vi "LCR_development_test.vi"() -> ()   [LabVIEW 2018]
uses:
  InstrControl/LCRControl/LCRControl.lvclass
  InstrControl/InstrControl.lvclass
panel:
  out "Resistance in Ohm":dbl
  out "Capacitance in pF":dbl
  out "Instrument name OUT":string
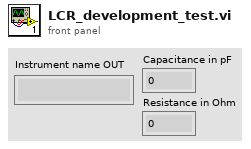
[diagram p1: front panel]
types:
  T1 = enum16{"Supply", "LCR", "Multimeter", "Switching"}
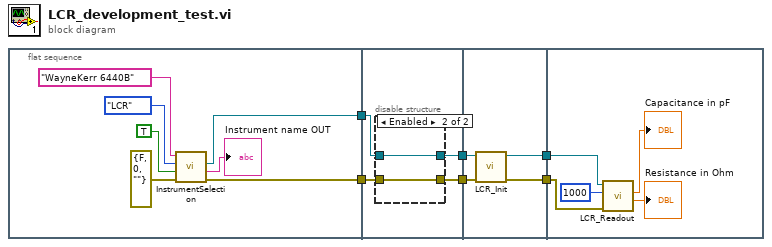
[diagram p0: block diagram]
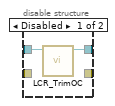
[diagram p2: hidden frame]
diagram:
  n1 = flat-sequence {
    tunnel: [w8] -> w6
    tunnel: [w7] -> w2
    tunnel: w6 -> [w17]
    tunnel: [w16] -> w5
    tunnel: [w15] -> w3
    tunnel: w2 -> [w14]
    tunnel: w5 -> [w25]
    tunnel: [w24] -> w4
    tunnel: w3 -> [w23]
    tunnel: [w22] -> w1
    tunnel: w4 -> [w30]
    tunnel: w1 -> [w29]
    frame #0 {
      n2 = call "InstrumentSelection.vi"("error in (no error)"=errorcluster {"status"=FALSE, "code"=0, "source"=""}, "Verify GPIB address"=TRUE, "Instrument type"=T1."LCR", "Instrument name IN"="WayneKerr 6440B") -> ("error out"=w7:errorcluster, "Instrument name OUT"=→"Instrument name OUT":string, "LCR"=w8:refnum<class "LCRControl.lvclass">)  [unwired: 2 in, 3 out]
    }
    frame #1 {
      n3 = disable-structure shown="Enabled" {
        disable-tunnel: w17 -> [w19 w21]
        disable-tunnel: [w18 w21] -> w16
        disable-tunnel: [_ w20] -> w15
        disable-tunnel: w14 -> [_ w20]
        frame Disabled {
          n4 = call-dynamic "LCR_TrimOC.vi"("LCRControl in"=w19) -> ("LCRControl out"=w18:refnum<class "LCRControl.lvclass">)  [unwired: 9 in, 1 out]
        }
        frame Enabled {
        }
      }
    }
    frame #2 {
      n5 = call-dynamic "LCR_Init.vi"("error in (no error)"=w23, "LCRControl in"=w25) -> ("error out"=w22:errorcluster, "LCRControl out"=w24:refnum<class "LCRControl.lvclass">)  [unwired: 8 in]
    }
    frame #3 {
      n6 = call-dynamic "LCR_Readout.vi"("error in (no error)"=w29, "Frequency in Hz"=1000, "LCRControl in"=w30) -> ("Resistance in Ohm"=→"Resistance in Ohm":dbl, "Capacitance in pF"=→"Capacitance in pF":dbl)  [unwired: 5 in, 2 out]
    }
  }
